vi "Read IQ Recorder Measurement IQ Data.vi"(8 "error in (no error)":errorcluster, 9 "Instance (1)":i32=1, 11 "VISA resource name":refnum<visa-resource-name>) -> (0 "error out":errorcluster, 1 "Q Amplitudes":dbl[](array[numeric]) format="%^.3e", 2 "I Amplitudes":dbl[](array[numeric]) format="%^.3e", 3 "VISA resource name out":refnum<visa-resource-name>)   [LabVIEW 2020, in "Rohde&Schwarz CMXP GPRF.lvlib"]
doc: "Returns I/Q recorder results in binary format.\n\nAttribute:\nRSCMXPGPRF_ATTR_READ_IQ_RECORDER_BIN_DATA\n\nRemote-control command:\nREAD:GPRF:MEAS<i>:IQRecorder:BIN?"
uses:
  <instrlib>/Rohde&Schwarz CMXP GPRF/Rohde&Schwarz CMXP GPRF.lvlib
  <instrlib>/Rohde&Schwarz CMXP GPRF/Private/rsidr_core.llb/type_Binary_Float_Number_Format.ctl
  <instrlib>/Rohde&Schwarz CMXP GPRF/Private/rsidr_core.llb/rsidr_core.lvlib
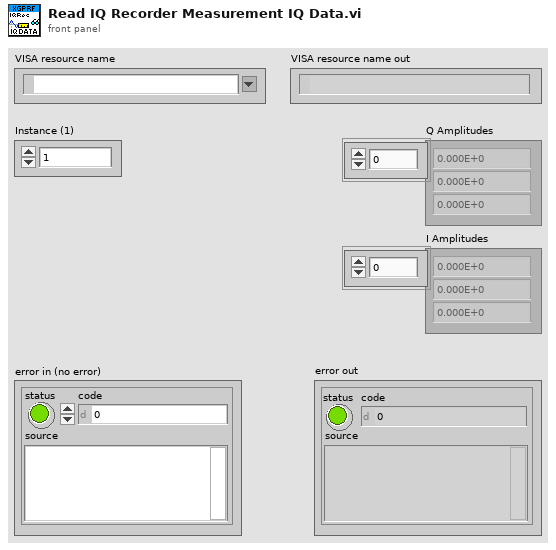
[diagram p1: front panel]
types:
  T1 = typedef "Rohde&Schwarz CMXP GPRF.lvlib/rsidr_core.lvlib/type_Binary_Float_Number_Format.ctl" = enum16{"Float_4_Bytes_Swapped", "Float_4_Bytes", "Double_8_Bytes_Swapped", "Double_8_Bytes"}
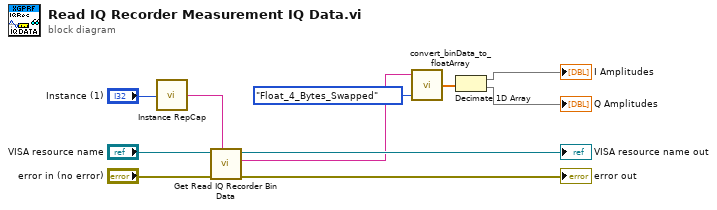
[diagram p0: block diagram]
diagram:
  n1 = call <instrlib>:"Instance RepCap.vi"("Instance in"="Instance (1)") -> ("Instance out"=w6:string)
  n2 = call "Get Read IQ Recorder Bin Data"("Repeated Capabilities"=w6, "error in (no error)"="error in (no error)", "instrument handle"="VISA resource name") -> ("error out"=→"error out":errorcluster, "Read IQ Recorder Bin Data"=w1:string, "instrument handle out"=→"VISA resource name out":refnum<visa-resource-name>)  [unwired: 6 in]
  n3 = call <instrlib>:"convert_binData_to_floatArray.vi"("Bin Float Number Format"=type_Binary_Float_Number_Format."Float_4_Bytes_Swapped", "Bin Data"=w1) -> ("Numbers out"=w4:dbl[])  [unwired: 1 in, 2 out]
  n4 = Decimate 1D Array(w4) -> (→"I Amplitudes":dbl[], →"Q Amplitudes":dbl[])
